vi "MeasureSet.vi"(7 "参数查询(0)/设置(1)":bool, 8 "error in (no error)":errorcluster caption="错误输入（无错误）", 9 "设置参数":string, 10 "MEASURE命令子系统":string(combo), 11 "VISA资源名称":refnum<visa-resource-name>) -> (0 "error out":errorcluster caption="错误输出", 1 "查询返回字节数":u32, 2 "查询返回":string, 3 "VISA资源名称 2":refnum<visa-resource-name>)   [LabVIEW 2018]
uses:
  <vilib>/regexp/Match Regular Expression.xnode
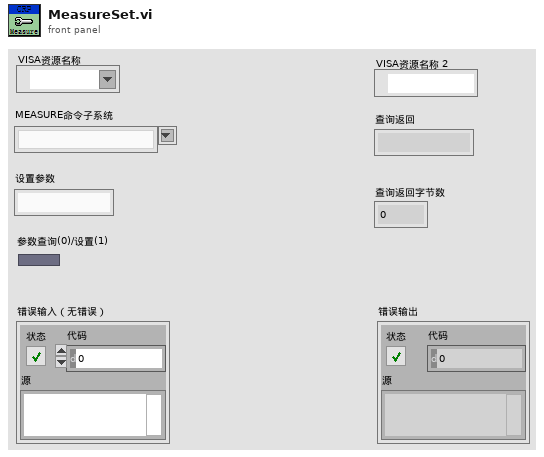
[diagram p1: front panel]
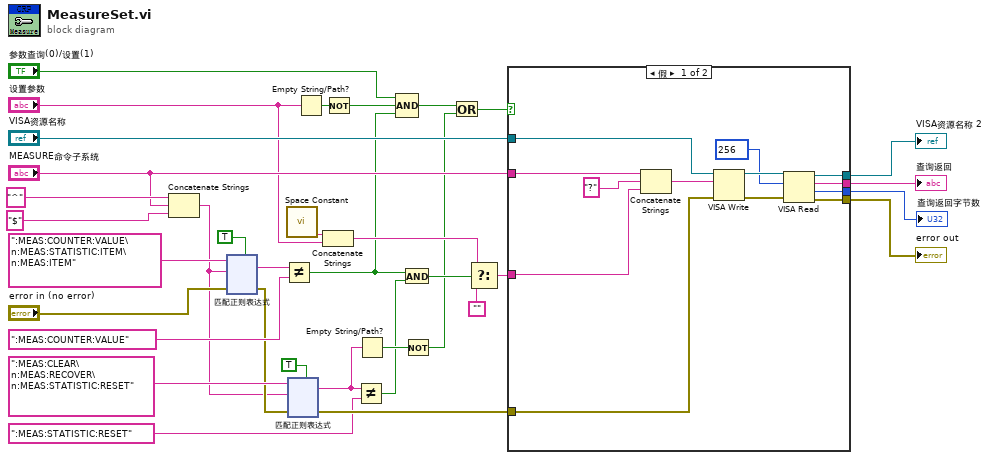
[diagram p0: block diagram]
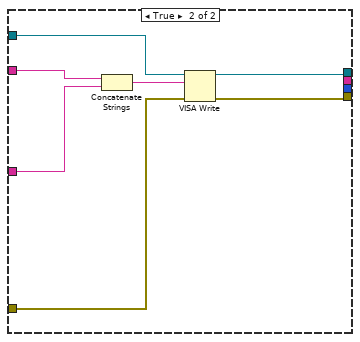
[diagram p2: hidden frame]
diagram:
  n1 = Concatenate Strings("^" ("字符串"), "MEASURE命令子系统", "$" ("字符串")) -> (w11:string)
  n2 = xnode "匹配正则表达式"("输入字符串"=":MEAS:COUNTER:VALUE\n:MEAS:STATISTIC:ITEM\n:MEAS:ITEM", "正则表达式"=w11, "错误输入"="error in (no error)", "多行？<B><B>(F)</B></B>"=TRUE) -> ("所有匹配"=w21:string, "错误输出"=w13:errorcluster)  [unwired: 2 in, 3 out]
  n3 = Not Equal?(x=w21, y=":MEAS:COUNTER:VALUE") -> (x != y?=w5:bool)
  n4 = call <vilib>:"Space Constant.vi"() -> ("String"=w27:string)
  n5 = xnode "匹配正则表达式"("输入字符串"=":MEAS:CLEAR\n:MEAS:RECOVER\n:MEAS:STATISTIC:RESET", "正则表达式"=w11, "错误输入"=w13, "多行？<B><B>(F)</B></B>"=TRUE) -> ("所有匹配"=w4:string, "错误输出"=w12:errorcluster)  [unwired: 2 in, 3 out]
  n6 = Empty String/Path?(string/path="设置参数") -> (empty?=w31:bool)
  n7 = Concatenate Strings(w27, "设置参数") -> (w18:string)
  n8 = Not(x=w31) -> (.not. x?=w28:bool)
  n9 = Not Equal?(x=w4, y=":MEAS:STATISTIC:RESET") -> (x != y?=w1:bool)
  n10 = Empty String/Path?(string/path=w4) -> (empty?=w3:bool)
  n11 = Compound Arithmetic op=AND ("复合运算")("参数查询(0)/设置(1)", w28, w5) -> (w9:bool)
  n12 = And(x=w5, y=w1) -> (x .and. y?=w6:bool)
  n13 = Not(x=w3) -> (.not. x?=w2:bool)
  n14 = Or(x=w9, y=w2) -> (x .or. y?=w10:bool)
  n15 = Select(t=w18, s=w6, f="") -> (s? t:f=w17:string)
  n16 = case shown="假" w10 {
    tunnel: "MEASURE命令子系统" -> [w48 w55]
    tunnel: "VISA资源名称" -> [w45 w54]
    tunnel: w12 -> [w44 w52]
    tunnel: [w40 w50] -> w32
    tunnel: [w39 w51] -> w33
    tunnel: [w38 _] -> w34
    tunnel: [w37 _] -> w29
    tunnel: w17 -> [w36 w49]
    frame False {
      n17 = Concatenate Strings(w48, "?" ("字符串"), w36) -> (w46:string)
      n18 = VISA Write(VISA resource name=w45, write buffer=w46, error in (no error)=w44) -> (VISA resource name out=w43:refnum<visa-resource-name>, error out=w42:errorcluster)  [unwired: 1 out]
      n19 = VISA Read(VISA resource name=w43, byte count=u32 256 ("字节总数"), error in (no error)=w42) -> (VISA resource name out=w39:refnum<visa-resource-name>, read buffer=w38:string, return count=w37:u32, error out=w40:errorcluster)
    }
    frame True {
      n20 = Concatenate Strings(w55, w49) -> (w53:string)
      n21 = VISA Write(VISA resource name=w54, write buffer=w53, error in (no error)=w52) -> (VISA resource name out=w51:refnum<visa-resource-name>, error out=w50:errorcluster)  [unwired: 1 out]
    }
  }
  "VISA资源名称 2" <- w33
  "error out" <- w32
  "查询返回" <- w34
  "查询返回字节数" <- w29
